vi "disable.vi"(0 "Return To Home Position":bool, 1 "Exit":bool, 2 "Rooms":i32(slide) scale=1.0..8.0, 3 "Do You Want To Clean The LivingRoom?":bool, 4 "X":dbl min=-200.0 max=200.0 step=1.0, 5 "Y":dbl min=-200.0 max=200.0 step=1.0) -> ()   [LabVIEW 2013]
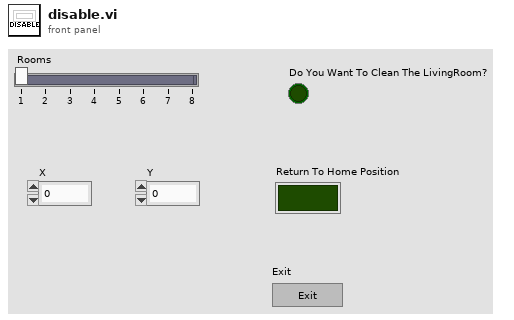
[diagram p1: front panel]
types:
  T1 = enum8{"Enabled", "Disabled", "Disabled and Grayed Out"}
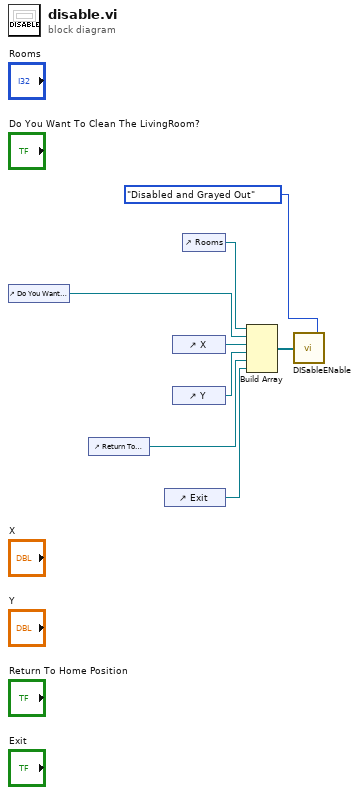
[diagram p0: block diagram]
diagram:
  n1 = control-ref of="Do You Want To Clean The LivingRoom?"() -> (w7:refnum<vi>)
  n2 = control-ref of="Return To Home Position"() -> (w4:refnum<vi>)
  n3 = control-ref of="Exit"() -> (w3:refnum<vi>)
  n4 = control-ref of="X"() -> (w6:refnum<vi>)
  n5 = control-ref of="Y"() -> (w5:refnum<vi>)
  n6 = control-ref of="Rooms"() -> (w8:refnum<vi>)
  n7 = Build Array(w8, w7, w6, w5, w4, w3) -> (w1:refnum<vi>[])
  n8 = call "DISableENable.vi"("Disabled"=T1."Disabled and Grayed Out", "Array"=w1) -> ()
